vi "ЛР5 - 1 варик - копия.vi"() -> ()   [LabVIEW 2012]
uses:
  <vilib>/Analysis/3filter.llb/Filter Passband Type.ctl
  <vilib>/Analysis/_algsub.llb/Vector Norm Type.ctl
  <vilib>/Analysis/2dsp.llb/1D Auto Correlation (DBL).vi
  <vilib>/Analysis/baseanly.llb/Normalize Vector.vi
  <vilib>/Analysis/baseanly.llb/Unit Vector (DBL).vi
  <vilib>/Analysis/3filter.llb/Chebyshev Filter (DBL).vi
  <vilib>/Analysis/3filter.llb/Butterworth Filter (DBL).vi
  <vilib>/Analysis/NI_AALBase.lvlib
  <vilib>/Analysis/NI_AALPro.lvlib
  <vilib>/Analysis/NI_AAL_SigProc.lvlib
panel:
  in  "stop":bool
  in  "Ring":u16(ring) items=["Chebishev", "Butterworth Filter"]
  out "Autocorrelation":dbl[](graph)
  out "mean":dbl format="%0.2f"
  out "standard deviation":dbl format="%0.2f"
  out "Normalize Vector":dbl[](graph)
  out "Unit Vector":dbl[](graph)
  out "norm":dbl format="%0.2f"
  in  "norm type":T1=2 items=["1-norm"=1, "2-norm"=2, "Inf-norm"=3, "-Inf-norm"=4, "User Defined"=5]
  in  "threshold":dbl format="%0.2f"
  in  "width":i32=3 min=3
  out "Locations 2":dbl[](array[numeric])
  out "# found 2":i32
  out "2nd Derivatives 2":dbl[](array[numeric])
  out "Amplitudes 3":dbl[](array[numeric])
  out "Locations":dbl[](array[numeric])
  out "# found":i32
  out "2nd Derivatives":dbl[](array[numeric])
  out "Amplitudes 2":dbl[](array[numeric])
  out "DC estimate (V)":dbl format="%0.2f"
  out "AC estimate (Vrms)":dbl format="%0.2f"
  in  "Cluster 3":T3={"sampling freq: fs"=1.0, "high cutoff freq"=0.2, "low cutoff freq"=0.25, "order"=2, "ripple(dB)"=0.1, "filter type"=enum."Lowpass"} {"ripple(dB)" format="%0.2f"; "low cutoff freq" scale=0.0..10.0; "high cutoff freq" scale=0.0..10.0; "sampling freq: fs" scale=0.0..10.0}
  in  "Cluster 2":T4={"sampling freq: fs"=1.0, "high cutoff freq"=0.2, "low cutoff freq"=0.25, "order"=2, "filter type "=enum."Lowpass"} {"low cutoff freq" scale=0.0..10.0; "high cutoff freq" scale=0.0..10.0; "sampling freq: fs" scale=0.0..10.0}
  in  "Cluster":T5 {"Noise amplitude" scale=0.0..3.0; "Noise" items=["Uniform White", "Periodic Random", "Poisson Noise "]; "Sine frequency" scale=10.0..100.0; "Frequency" scale=0.0..10.0; "Amplitude" scale=0.0..10.0}
  out "Waveform Graph":dynamicdata(graph)
  # "Radio imp"
  # "Video imp"
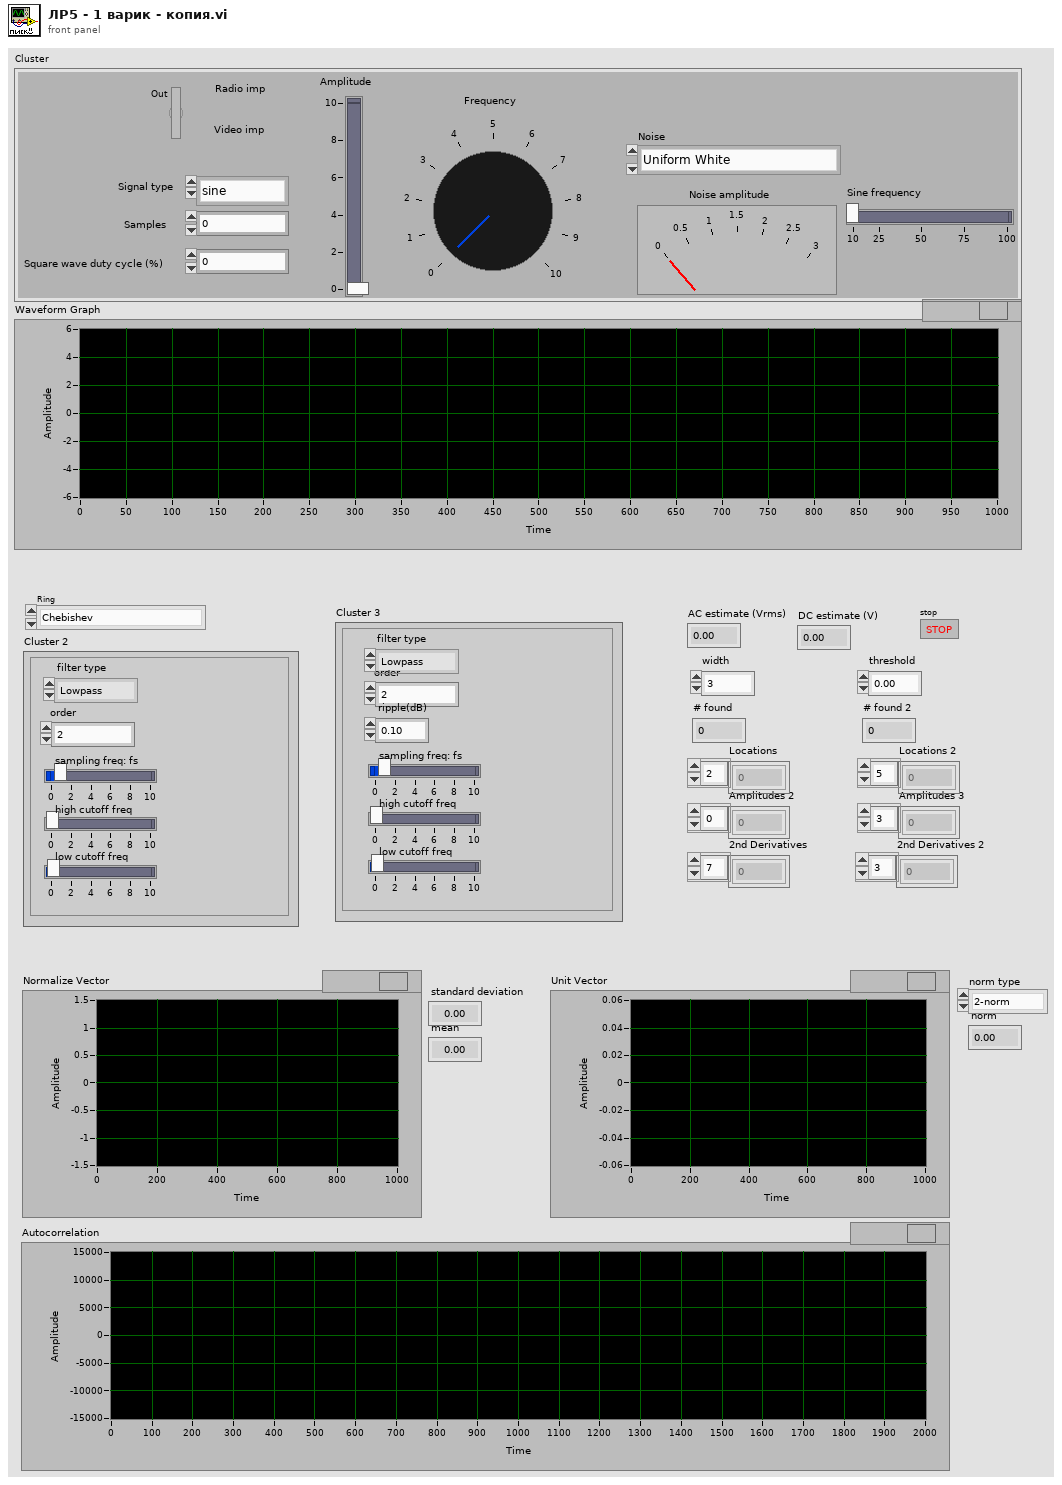
[diagram p1: front panel]
types:
  T1 = typedef "NI_AALPro.lvlib/Vector Norm Type.ctl" = u16
  T2 = typedef "NI_AALBase.lvlib/Filter Passband Type.ctl" = enum32{"Lowpass", "Highpass", "Bandpass", "Bandstop"}
  T3 = cluster{"sampling freq: fs":dbl, "high cutoff freq":dbl, "low cutoff freq":dbl, "order":i32, "ripple(dB)":dbl, "filter type":T2}
  T4 = cluster{"sampling freq: fs":dbl, "high cutoff freq":dbl, "low cutoff freq":dbl, "order":i32, "filter type ":T2}
  T5 = cluster{"Amplitude":dbl, "Frequency":dbl, "Sine frequency":dbl, "Square wave duty cycle (%)":dbl, "Noise":u16, "Samples":i32, "Signal type":enum16{"sine", "cosine", "triangle", "square", "sawtooth", "increasing ramp", "decreasing ramp"}, "Noise amplitude":dbl, "Out":bool}
  T6 = enum16{"sine", "cosine", "triangle", "square", "sawtooth", "increasing ramp", "decreasing ramp"}
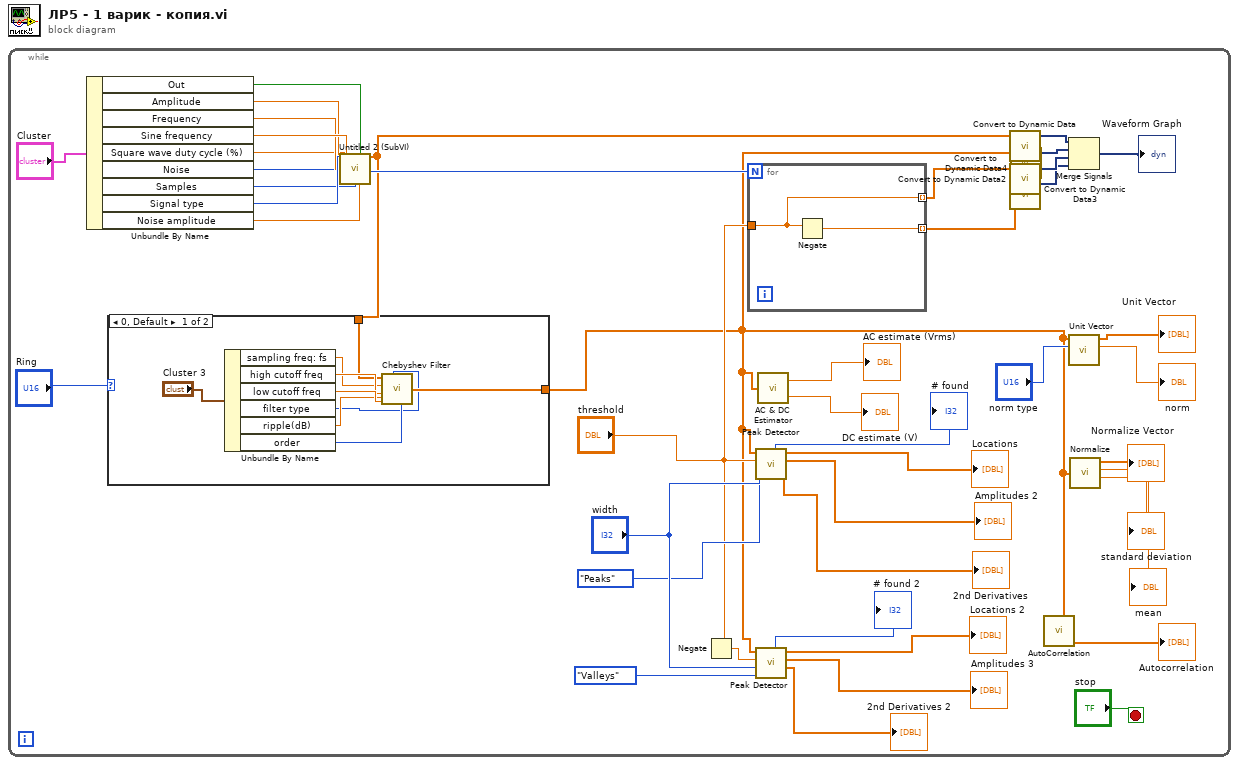
[diagram p0: block diagram]
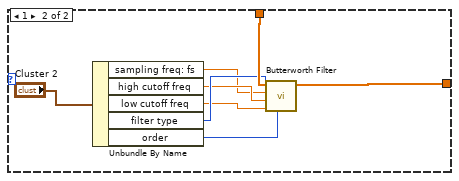
[diagram p2: hidden frame]
diagram:
  n1 = while {
    stop <- "stop" stop-if-true
    n2 = Unbundle By Name "Unbundle By Name"("Cluster") -> ("Out"=w13:bool, "Amplitude"=w9:dbl, "Frequency"=w10:dbl, "Sine frequency"=w11:dbl, "Square wave duty cycle (%)"=w7:dbl, "Noise"=w6:u16, "Samples"=w4:i32, "Signal type"=w12:T6, "Noise amplitude"=w8:dbl)
    n3 = call "Untitled 2 (SubVI).vi"("Signal type"=w12, "Sine frequency"=w11, "Samples"=w4, "Out"=w13, "Frequency"=w10, "Amplitude"=w9, "Square wave duty cycle (%)"=w7, "Noise"=w6, "Noise amplitude"=w8) -> ("Waveform Graph"=w2:dbl[])  [unwired: 6 in]
    n4 = case shown="0, Default" "Ring" {
      tunnel: [w48 w61] -> w3
      tunnel: w2 -> [w46 w60]
      frame 0, Default {
        n5 = Unbundle By Name("Cluster 3") -> ("sampling freq: fs"=w51:dbl, "high cutoff freq"=w52:dbl, "low cutoff freq"=w53:dbl, "filter type"=w47:T2, "ripple(dB)"=w49:dbl, "order"=w50:i32)
        n6 = call-poly <vilib>:"Chebyshev Filter.vi"("order"=w50, "ripple(dB)"=w49, "filter type"=w47, "low cutoff freq: fl"=w53, "high cutoff freq: fh"=w52, "sampling freq: fs"=w51, "X"=w46) -> ("Filtered X"=w48:dbl[])  [unwired: 3 in, 1 out]
      }
      frame 1 {
        n7 = Unbundle By Name("Cluster 2") -> ("sampling freq: fs"=w55:dbl, "high cutoff freq"=w56:dbl, "low cutoff freq"=w57:dbl, "filter type"=w59:T2, "order"=w58:i32)
        n8 = call-poly <vilib>:"Butterworth Filter.vi"("order"=w58, "filter type"=w59, "low cutoff freq: fl"=w57, "high cutoff freq: fh"=w56, "sampling freq: fs"=w55, "X"=w60) -> ("Filtered X"=w61:dbl[])  [unwired: 2 in, 1 out]
      }
    }
    n9 = Negate(x="threshold") -> (-x=w30:dbl)
    n10 = for {
      N: w4 -> [_]
      tunnel: "threshold" -> [w44]
      tunnel: [w45] -> w24 mode=indexing
      tunnel: [w44] -> w26 mode=indexing
      n11 = Negate(x=w44) -> (-x=w45:dbl)
    }
    n12 = call <vilib>:"Peak Detector.vi"("peaks/valleys"=enum32{"Peaks", "Valleys"}."Peaks", "width"="width", "threshold"="threshold", "X"=w3) -> ("2nd Derivatives"=→"2nd Derivatives":dbl[], "Amplitudes"=→"Amplitudes 2":dbl[], "Locations"=→"Locations":dbl[], "# found"=→"# found":i32)  [unwired: 3 in, 1 out]
    n13 = call <vilib>:"Peak Detector.vi"("peaks/valleys"=enum32{"Peaks", "Valleys"}."Valleys", "width"="width", "threshold"=w30, "X"=w3) -> ("2nd Derivatives"=→"2nd Derivatives 2":dbl[], "Amplitudes"=→"Amplitudes 3":dbl[], "Locations"=→"Locations 2":dbl[], "# found"=→"# found 2":i32)  [unwired: 3 in, 1 out]
    n14 = call <vilib>:"AC & DC Estimator.vi"("Signal (V)"=w3) -> ("AC estimate (Vrms)"=→"AC estimate (Vrms)":dbl, "DC estimate (V)"=→"DC estimate (V)":dbl)
    n15 = call "Convert to Dynamic Data"("Array"=w2) -> ("Dynamic Data Type"=w27:dynamicdata)  [unwired: 3 in]
    n16 = call "Convert to Dynamic Data2"("Array"=w26) -> ("Dynamic Data Type"=w25:dynamicdata)  [unwired: 3 in]
    n17 = call "Convert to Dynamic Data3"("Array"=w24) -> ("Dynamic Data Type"=w23:dynamicdata)  [unwired: 3 in]
    n18 = call "Convert to Dynamic Data4"("Array"=w3) -> ("Dynamic Data Type"=w22:dynamicdata)  [unwired: 3 in]
    n19 = call-poly <vilib>:"AutoCorrelation.vi"("X"=w3) -> ("Rxx"=→"Autocorrelation":dbl[])  [unwired: 9 in, 1 out]
    n20 = Merge Signals "Merge Signals"(w27, w22, w25, w23) -> (→"Waveform Graph":dynamicdata)
    n21 = call-poly <vilib>:"Unit Vector.vi"("norm type"="norm type", "Input Vector"=w3) -> ("norm"=→"norm":dbl, "Unit Vector"=→"Unit Vector":dbl[])  [unwired: 7 in, 1 out]
    n22 = call-poly <vilib>:"Normalize.vi"("Vector"=w3) -> ("mean"=→"mean":dbl, "standard deviation"=→"standard deviation":dbl, "Normalized Vector"=→"Normalize Vector":dbl[])  [unwired: 1 in, 1 out]
  }
